vi "_Configure Window.vi"(4 "For Printing (T)":bool=TRUE, 6 "Expt#":i32=1, 7 "ControlRef":T1) -> ()   [LabVIEW 2015]
uses:
  Type/_Run Module.ctl
  Type/_Data Operation.ctl
  Configuration/_Global Configuration.vi
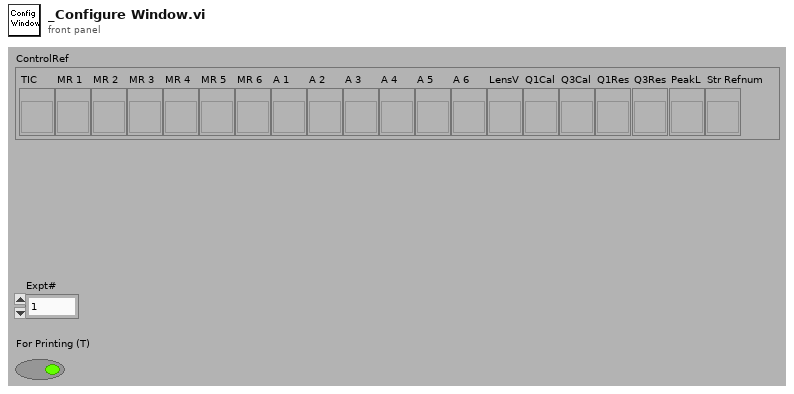
[diagram p1: front panel]
types:
  T1 = cluster{"TIC":refnum<vi>, "MR 1":refnum<vi>, "MR 2":refnum<vi>, "MR 3":refnum<vi>, "MR 4":refnum<vi>, "MR 5":refnum<vi>, "MR 6":refnum<vi>, "A 1":refnum<vi>, "A 2":refnum<vi>, "A 3":refnum<vi>, "A 4":refnum<vi>, "A 5":refnum<vi>, "A 6":refnum<vi>, "LensV":refnum<vi>, "Q1Cal":refnum<vi>, "Q3Cal":refnum<vi>, "Q1Res":refnum<vi>, "Q3Res":refnum<vi>, "PeakL":refnum<vi>, "Str Refnum":refnum<vi>}
  T2 = typedef "_Run Module.ctl" = u16
  T3 = typedef "_Data Operation.ctl" = enum8{"Initialize", "Get Data", "Set Data", "Close"}
  T4 = typedef "_Lens Property.ctl" = cluster{"Scan Type":u8, "Scans":i32, "Time 1":dbl, "Time 2":dbl, "Value 1":dbl, "Value 2":dbl, "Step Size":dbl}
  T5 = typedef "_Mass Range Property.ctl" = cluster{"Start":dbl, "Stop":dbl, "Step Size":dbl, "Steps":i32, "Dwell":dbl, "Parameters":T6[], "Res":T7}
  T6 = typedef "_Mass Range Parameters.ctl" = cluster{"Name":string, "Ch#":u8, "StartV":dbl, "StopV":dbl, "StepV":dbl, "Index":u8}
  T7 = typedef "_RT Res Type.ctl" = u16
  T8 = typedef "_Run Mode.ctl" = enum16{"MRM (Q1/Q2)", "Q1 Scan", "Q1 SRM", "Q2 Scan", "Q2 SRM", "Product Scan", "Precursor Scan", "Neutral Loss", "Neutral Gain"}
  T9 = cluster{"Lenses":T4[], "Mass Ranges":T5[], "Acquire":bool, "MCA":bool, "Q1DC EN":bool, "Q1 POL":bool, "Q3 POL":bool, "Q1 RF  EN":bool, "Averaging":bool, "Log Scale":bool, "CPS":bool, "Unit":bool, "Data Path":path, "Run Mode":T8, "Fixed Mass (amu)":dbl, "Q3DC EN":bool, "Q3 RF  EN":bool, "Negative":bool}
  T10 = typedef "_Current Data.ctl" = cluster{"Scan#":i32, "Run Time (mS)":i32, "TIC X":dbl[], "TIC Y":dbl[][], "MassRange":cluster{"X Title":string, "X":dbl[], "Y":i32[]}[], "Fixed Mass (amu)":dbl, "Method":T11}
  T11 = typedef "_XML Expt.ctl" = cluster{"StartT(mS)":i32, "#Cycles":i32, "PauseT(uS)":i32, "ScanType":i32, "Polarity":u8, "FixedMass":dbl, "DelayT(mS)":i32, "Active Ch":T12[], "Mass Range":T5[]}
  T12 = typedef "_XML Lens.ctl" = cluster{"Value":dbl, "ChID":u8}
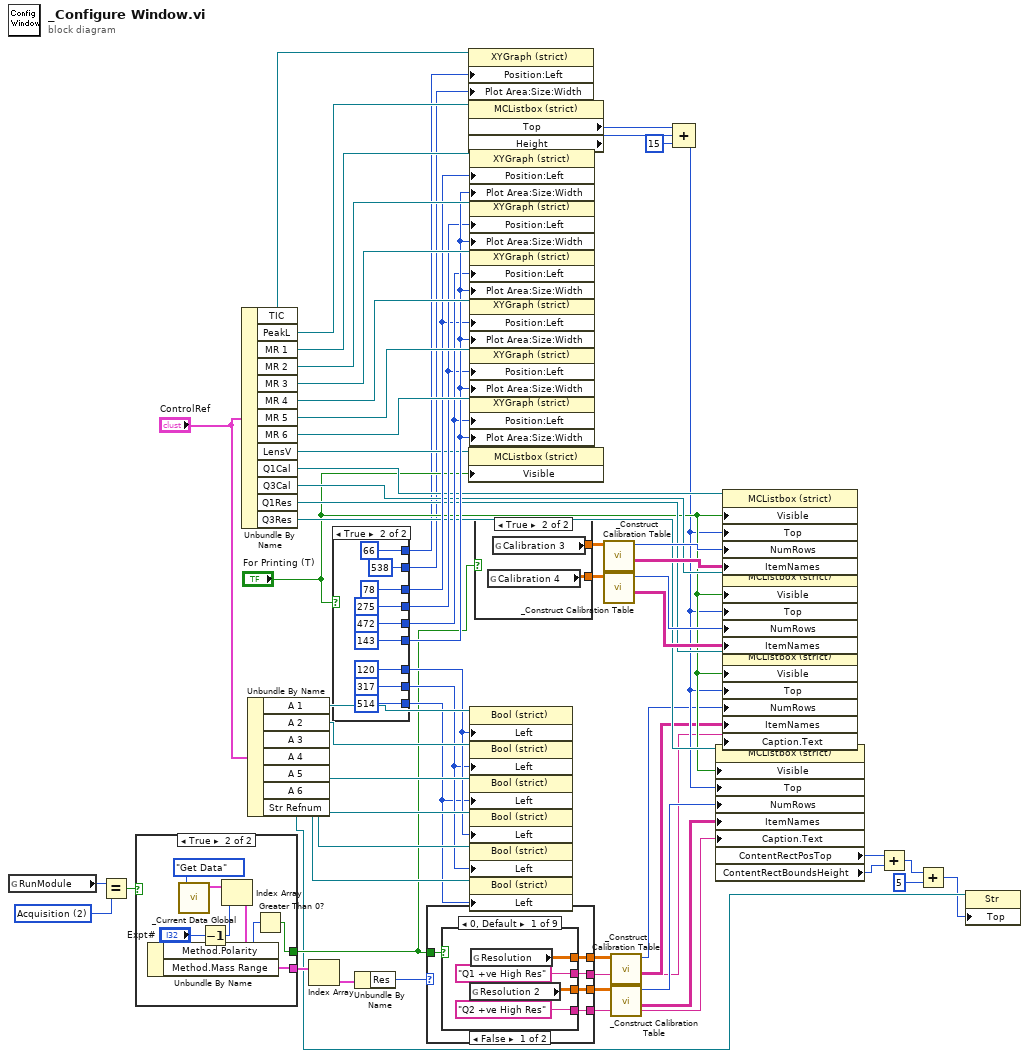
[diagram p0: block diagram]
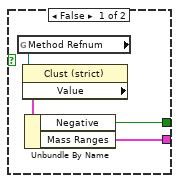
[diagram p2: hidden frame]
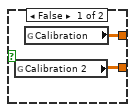
[diagram p3: hidden frame]
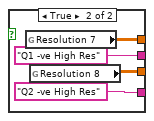
[diagram p4: hidden frame]
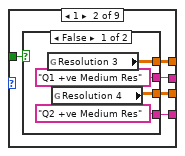
[diagram p5: hidden frame]
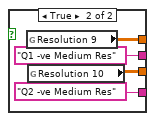
[diagram p6: hidden frame]
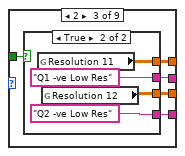
[diagram p7: hidden frame]
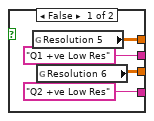
[diagram p8: hidden frame]
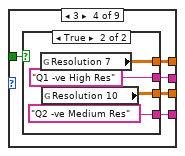
[diagram p9: hidden frame]
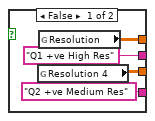
[diagram p10: hidden frame]
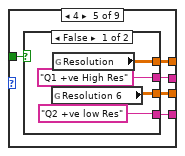
[diagram p11: hidden frame]
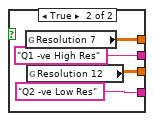
[diagram p12: hidden frame]
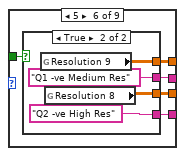
[diagram p13: hidden frame]
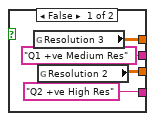
[diagram p14: hidden frame]
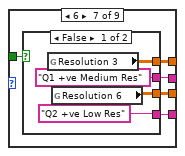
[diagram p15: hidden frame]
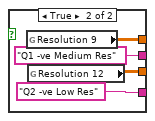
[diagram p16: hidden frame]
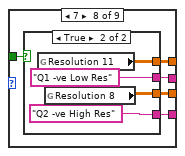
[diagram p17: hidden frame]
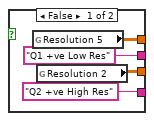
[diagram p18: hidden frame]
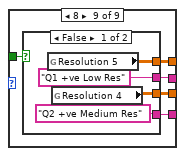
[diagram p19: hidden frame]
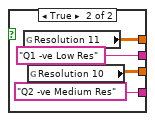
[diagram p20: hidden frame]
diagram:
  w12 = T2 2 items=["Diagnostics", "Tune", "Acquisition"] ("y")
  n1 = global read "_Global Configuration.vi" "RunModule"() -> (w13:T2)
  n2 = Equal?(x=w13, y=w12) -> (x = y?=w11:bool)
  n3 = case shown="True" w11 {
    tunnel: [w63 w69] -> w21
    tunnel: [w62 w68] -> w14
    frame False {
      n4 = global read "_Global Configuration.vi" "Method Refnum"() -> (w65:refnum<vi>)
      n5 = property class="Clust (strict)"(reference=w65) -> ("Value"=w64:T9)  [unwired: 1 in, 2 out]
      n6 = Unbundle By Name(w64) -> ("Negative"=w62:bool, "Mass Ranges"=w63:T5[])
    }
    frame True {
      n7 = call "_Current Data Global.vi"("Operation"=_Data_Operation."Get Data") -> ("CurrentData"=w72:T10[])  [unwired: 3 in, 3 out]
      n8 = Decrement(x="Expt#") -> (x-1=w66:i32)
      n9 = Index Array(array=w72, index=w66) -> (element=w70:T10)
      n10 = Unbundle By Name(w70) -> ("Method.Polarity"=w67:u8, "Method.Mass Range"=w69:T5[])
      n11 = Greater Than 0?(x=w67) -> (x > 0?=w68:bool)
    }
  }
  n12 = Unbundle By Name("ControlRef") -> ("TIC"=w9:refnum<vi>, "PeakL"=w41:refnum<vi>, "MR 1"=w61:refnum<vi>, "MR 2"=w59:refnum<vi>, "MR 3"=w58:refnum<vi>, "MR 4"=w57:refnum<vi>, "MR 5"=w56:refnum<vi>, "MR 6"=w60:refnum<vi>, "LensV"=w51:refnum<vi>, "Q1Cal"=w40:refnum<vi>, "Q3Cal"=w33:refnum<vi>, "Q1Res"=w29:refnum<vi>, "Q3Res"=w28:refnum<vi>)
  n13 = Unbundle By Name("ControlRef") -> ("A 1"=w50:refnum<vi>, "A 2"=w49:refnum<vi>, "A 3"=w48:refnum<vi>, "A 4"=w47:refnum<vi>, "A 5"=w46:refnum<vi>, "A 6"=w45:refnum<vi>, "Str Refnum"=w4:refnum<vi>)
  n14 = Index Array(array=w21) -> (element=w20:T5)  [unwired: 1 in]
  n15 = case shown="True" "For Printing (T)" {
    tunnel: [-52 ("Position:Left") 78 ("Position:Left")] -> w52
    tunnel: [189 ("Plot Area:Size:Width") 275 ("Plot Area:Size:Width")] -> w53
    tunnel: [429 ("Plot Area:Size:Width") 472 ("Plot Area:Size:Width")] -> w54
    tunnel: [u32 186 ("Plot Area:Size:Width") u32 143 ("Plot Area:Size:Width")] -> w55
    tunnel: [-10 ("Position:Left") 120 ("Position:Left")] -> w44
    tunnel: [231 ("Plot Area:Size:Width") 317 ("Plot Area:Size:Width")] -> w43
    tunnel: [471 ("Plot Area:Size:Width") 514 ("Plot Area:Size:Width")] -> w42
    tunnel: [-64 ("Position:Left") 66 ("Position:Left")] -> w8
    tunnel: [u32 668 ("Plot Area:Size:Width") u32 538 ("Plot Area:Size:Width")] -> w7
    frame False {
    }
    frame True {
    }
  }
  n16 = Unbundle By Name(w20) -> ("Res"=w19:T7)
  n17 = case shown="0, Default" w19 {
    tunnel: [w96 w109 w122 w135 w148 w161 w174 w187 w200] -> w18
    tunnel: [w95 w108 w121 w134 w147 w160 w173 w186 w199] -> w17
    tunnel: [w94 w107 w120 w133 w146 w159 w172 w185 w198] -> w16
    tunnel: [w93 w106 w119 w132 w145 w158 w171 w184 w197] -> w15
    tunnel: w14 -> [w92 w105 w118 w131 w144 w157 w170 w183 w196]
    frame 0, Default {
      n18 = case shown="False" w92 {
        tunnel: [w100 w104] -> w96
        tunnel: [w99 w102] -> w95
        tunnel: ["Q1 +ve High Res" "Q1 -ve High Res"] -> w94
        tunnel: ["Q2 +ve High Res" "Q2 -ve High Res"] -> w93
        frame False {
          n19 = global read "_Global Configuration.vi" "Resolution 2"() -> (w99:dbl[][])
          n20 = global read "_Global Configuration.vi" "Resolution"() -> (w100:dbl[][])
        }
        frame True {
          n21 = global read "_Global Configuration.vi" "Resolution 7"() -> (w104:dbl[][])
          n22 = global read "_Global Configuration.vi" "Resolution 8"() -> (w102:dbl[][])
        }
      }
    }
    frame 1 {
      n23 = case shown="False" w105 {
        tunnel: [w113 w117] -> w109
        tunnel: [w112 w115] -> w108
        tunnel: ["Q1 +ve Medium Res" "Q1 -ve Medium Res"] -> w107
        tunnel: ["Q2 +ve Medium Res" "Q2 -ve Medium Res"] -> w106
        frame False {
          n24 = global read "_Global Configuration.vi" "Resolution 3"() -> (w113:dbl[][])
          n25 = global read "_Global Configuration.vi" "Resolution 4"() -> (w112:dbl[][])
        }
        frame True {
          n26 = global read "_Global Configuration.vi" "Resolution 9"() -> (w117:dbl[][])
          n27 = global read "_Global Configuration.vi" "Resolution 10"() -> (w115:dbl[][])
        }
      }
    }
    frame 2 {
      n28 = case shown="True" w118 {
        tunnel: [w126 w130] -> w122
        tunnel: [w125 w128] -> w121
        tunnel: ["Q1 +ve Low Res" "Q1 -ve Low Res"] -> w120
        tunnel: ["Q2 +ve Low Res" "Q2 -ve Low Res"] -> w119
        frame False {
          n29 = global read "_Global Configuration.vi" "Resolution 5"() -> (w126:dbl[][])
          n30 = global read "_Global Configuration.vi" "Resolution 6"() -> (w125:dbl[][])
        }
        frame True {
          n31 = global read "_Global Configuration.vi" "Resolution 11"() -> (w130:dbl[][])
          n32 = global read "_Global Configuration.vi" "Resolution 12"() -> (w128:dbl[][])
        }
      }
    }
    frame 3 {
      n33 = case shown="True" w131 {
        tunnel: [w139 w143] -> w135
        tunnel: [w138 w141] -> w134
        tunnel: ["Q1 +ve High Res" "Q1 -ve High Res"] -> w133
        tunnel: ["Q2 +ve Medium Res" "Q2 -ve Medium Res"] -> w132
        frame False {
          n34 = global read "_Global Configuration.vi" "Resolution 4"() -> (w138:dbl[][])
          n35 = global read "_Global Configuration.vi" "Resolution"() -> (w139:dbl[][])
        }
        frame True {
          n36 = global read "_Global Configuration.vi" "Resolution 7"() -> (w143:dbl[][])
          n37 = global read "_Global Configuration.vi" "Resolution 10"() -> (w141:dbl[][])
        }
      }
    }
    frame 4 {
      n38 = case shown="False" w144 {
        tunnel: [w152 w156] -> w148
        tunnel: [w151 w154] -> w147
        tunnel: ["Q1 +ve High Res" "Q1 -ve High Res"] -> w146
        tunnel: ["Q2 +ve low Res" "Q2 -ve Low Res"] -> w145
        frame False {
          n39 = global read "_Global Configuration.vi" "Resolution 6"() -> (w151:dbl[][])
          n40 = global read "_Global Configuration.vi" "Resolution"() -> (w152:dbl[][])
        }
        frame True {
          n41 = global read "_Global Configuration.vi" "Resolution 7"() -> (w156:dbl[][])
          n42 = global read "_Global Configuration.vi" "Resolution 12"() -> (w154:dbl[][])
        }
      }
    }
    frame 5 {
      n43 = case shown="True" w157 {
        tunnel: [w165 w169] -> w161
        tunnel: [w164 w167] -> w160
        tunnel: ["Q1 +ve Medium Res" "Q1 -ve Medium Res"] -> w159
        tunnel: ["Q2 +ve High Res" "Q2 -ve High Res"] -> w158
        frame False {
          n44 = global read "_Global Configuration.vi" "Resolution 3"() -> (w165:dbl[][])
          n45 = global read "_Global Configuration.vi" "Resolution 2"() -> (w164:dbl[][])
        }
        frame True {
          n46 = global read "_Global Configuration.vi" "Resolution 9"() -> (w169:dbl[][])
          n47 = global read "_Global Configuration.vi" "Resolution 8"() -> (w167:dbl[][])
        }
      }
    }
    frame 6 {
      n48 = case shown="False" w170 {
        tunnel: [w178 w182] -> w174
        tunnel: [w177 w180] -> w173
        tunnel: ["Q1 +ve Medium Res" "Q1 -ve Medium Res"] -> w172
        tunnel: ["Q2 +ve Low Res" "Q2 -ve Low Res"] -> w171
        frame False {
          n49 = global read "_Global Configuration.vi" "Resolution 3"() -> (w178:dbl[][])
          n50 = global read "_Global Configuration.vi" "Resolution 6"() -> (w177:dbl[][])
        }
        frame True {
          n51 = global read "_Global Configuration.vi" "Resolution 9"() -> (w182:dbl[][])
          n52 = global read "_Global Configuration.vi" "Resolution 12"() -> (w180:dbl[][])
        }
      }
    }
    frame 7 {
      n53 = case shown="True" w183 {
        tunnel: [w191 w195] -> w187
        tunnel: [w190 w193] -> w186
        tunnel: ["Q1 +ve Low Res" "Q1 -ve Low Res"] -> w185
        tunnel: ["Q2 +ve High Res" "Q2 -ve High Res"] -> w184
        frame False {
          n54 = global read "_Global Configuration.vi" "Resolution 5"() -> (w191:dbl[][])
          n55 = global read "_Global Configuration.vi" "Resolution 2"() -> (w190:dbl[][])
        }
        frame True {
          n56 = global read "_Global Configuration.vi" "Resolution 11"() -> (w195:dbl[][])
          n57 = global read "_Global Configuration.vi" "Resolution 8"() -> (w193:dbl[][])
        }
      }
    }
    frame 8 {
      n58 = case shown="False" w196 {
        tunnel: [w204 w208] -> w200
        tunnel: [w203 w206] -> w199
        tunnel: ["Q1 +ve Low Res" "Q1 -ve Low Res"] -> w198
        tunnel: ["Q2 +ve Medium Res" "Q2 -ve Medium Res"] -> w197
        frame False {
          n59 = global read "_Global Configuration.vi" "Resolution 5"() -> (w204:dbl[][])
          n60 = global read "_Global Configuration.vi" "Resolution 4"() -> (w203:dbl[][])
        }
        frame True {
          n61 = global read "_Global Configuration.vi" "Resolution 11"() -> (w208:dbl[][])
          n62 = global read "_Global Configuration.vi" "Resolution 10"() -> (w206:dbl[][])
        }
      }
    }
  }
  n63 = property class="XYGraph (strict)"(reference=w9, "Position:Left"=w8, "Plot Area:Size:Width"=w7) -> ()  [unwired: 1 in, 2 out]
  n64 = property class="MCListbox (strict)"(reference=w41) -> ("Top"=w39:i32, "Height"=w38:u32)  [unwired: 1 in, 2 out]
  n65 = property class="MCListbox (strict)"(reference=w51, "Visible"="For Printing (T)") -> ()  [unwired: 1 in, 2 out]
  n66 = property class="XYGraph (strict)"(reference=w61, "Position:Left"=w52, "Plot Area:Size:Width"=w55) -> ()  [unwired: 1 in, 2 out]
  n67 = property class="XYGraph (strict)"(reference=w59, "Position:Left"=w53, "Plot Area:Size:Width"=w55) -> ()  [unwired: 1 in, 2 out]
  n68 = property class="XYGraph (strict)"(reference=w58, "Position:Left"=w54, "Plot Area:Size:Width"=w55) -> ()  [unwired: 1 in, 2 out]
  n69 = property class="XYGraph (strict)"(reference=w57, "Position:Left"=w52, "Plot Area:Size:Width"=w55) -> ()  [unwired: 1 in, 2 out]
  n70 = property class="XYGraph (strict)"(reference=w56, "Position:Left"=w53, "Plot Area:Size:Width"=w55) -> ()  [unwired: 1 in, 2 out]
  n71 = property class="XYGraph (strict)"(reference=w60, "Position:Left"=w54, "Plot Area:Size:Width"=w55) -> ()  [unwired: 1 in, 2 out]
  n72 = property class="Bool (strict)"(reference=w50, "Left"=w44) -> ()  [unwired: 1 in, 2 out]
  n73 = property class="Bool (strict)"(reference=w49, "Left"=w43) -> ()  [unwired: 1 in, 2 out]
  n74 = property class="Bool (strict)"(reference=w48, "Left"=w42) -> ()  [unwired: 1 in, 2 out]
  n75 = property class="Bool (strict)"(reference=w47, "Left"=w44) -> ()  [unwired: 1 in, 2 out]
  n76 = property class="Bool (strict)"(reference=w46, "Left"=w43) -> ()  [unwired: 1 in, 2 out]
  n77 = property class="Bool (strict)"(reference=w45, "Left"=w42) -> ()  [unwired: 1 in, 2 out]
  n78 = case shown="True" w14 {
    tunnel: [w210 w212] -> w36
    tunnel: [w209 w211] -> w32
    frame False {
      n79 = global read "_Global Configuration.vi" "Calibration 2"() -> (w209:dbl[][])
      n80 = global read "_Global Configuration.vi" "Calibration"() -> (w210:dbl[][])
    }
    frame True {
      n81 = global read "_Global Configuration.vi" "Calibration 4"() -> (w211:dbl[][])
      n82 = global read "_Global Configuration.vi" "Calibration 3"() -> (w212:dbl[][])
    }
  }
  n83 = call "_Construct Calibration Table.vi"("Calibration"=w36) -> ("Table"=w34:string[][], "Rows"=w35:i32)  [unwired: 5 out]
  n84 = call "_Construct Calibration Table.vi"("Calibration"=w32) -> ("Table"=w30:string[][], "Rows"=w31:i32)  [unwired: 5 out]
  n85 = call "_Construct Calibration Table.vi"("Calibration"=w18) -> ("Table"=w24:string[][], "Rows"=w25:i32)  [unwired: 5 out]
  n86 = call "_Construct Calibration Table.vi"("Calibration"=w17) -> ("Table"=w22:string[][], "Rows"=w23:i32)  [unwired: 5 out]
  n87 = Compound Arithmetic op=ADD(w39, w38, u32 15 ("value")) -> (w26:u32)
  n88 = property class="MCListbox (strict)"(reference=w28, "Visible"="For Printing (T)", "Top"=w26, "NumRows"=w23, "ItemNames"=w22, "Caption.Text"=w15) -> ("ContentRectPosTop"=w6:i32, "ContentRectBoundsHeight"=w5:i32)  [unwired: 1 in, 2 out]
  n89 = property class="MCListbox (strict)"(reference=w40, "Visible"="For Printing (T)", "Top"=w26, "NumRows"=w35, "ItemNames"=w34) -> ()  [unwired: 1 in, 2 out]
  n90 = property class="MCListbox (strict)"(reference=w33, "Visible"="For Printing (T)", "Top"=w26, "NumRows"=w31, "ItemNames"=w30) -> ()  [unwired: 1 in, 2 out]
  n91 = property class="MCListbox (strict)"(reference=w29, "Visible"="For Printing (T)", "Top"=w26, "NumRows"=w25, "ItemNames"=w24, "Caption.Text"=w16) -> ()  [unwired: 1 in, 2 out]
  n92 = Add(x=w6, y=w5) -> (x+y=w3:i32)
  n93 = Add(x=w3, y=5 ("x")) -> (x+y=w2:i32)
  n94 = property class="Str"(reference=w4, "Top"=w2) -> ()  [unwired: 1 in, 2 out]
